vi "Alignment Offset SLM.vi"() -> (3 "number of steps align":u16)   [LabVIEW 2014]
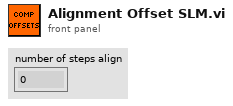
[diagram p1: front panel]
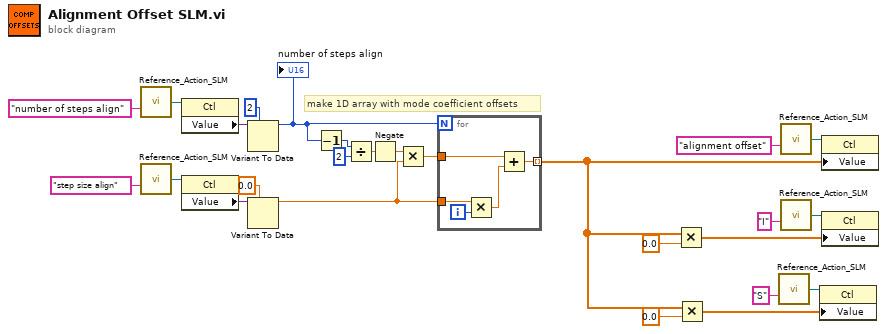
[diagram p0: block diagram]
diagram:
  # "make 1D array with mode coefficient offsets"
  n1 = call "Reference_Action_SLM.vi"("Control Name"="number of steps align") -> ("Ref OUT"=w15:refnum<vi>)  [unwired: 12 in, 2 out]
  n2 = call "Reference_Action_SLM.vi"("Control Name"="step size align") -> ("Ref OUT"=w20:refnum<vi>)  [unwired: 12 in, 2 out]
  n3 = property class="Ctl"(reference=w15) -> ("Value"=w16:variant)  [unwired: 1 in, 2 out]
  n4 = property class="Ctl"(reference=w20) -> ("Value"=w21:variant)  [unwired: 1 in, 2 out]
  n5 = Variant To Data(type=u16 2 ("y"), Variant=w16) -> (data=w12:u16)  [unwired: 1 in, 1 out]
  "number of steps align" <- w12
  n6 = Variant To Data(type=0.0 ("x*y"), Variant=w21) -> (data=w18:dbl)  [unwired: 1 in, 1 out]
  n7 = Decrement(x=w12) -> (x-1=w26:u16)
  n8 = Divide(x=w26, y=u16 2) -> (x/y=w24:dbl)
  n9 = Negate(x=w24) -> (-x=w25:dbl)
  n10 = Multiply(x=w25, y=w18) -> (x*y=w22:dbl)
  n11 = for {
    N: w12 -> [_]
    tunnel: w18 -> [w29]
    tunnel: w22 -> [w31]
    tunnel: [w27] -> w3 mode=indexing
    i -> [w30]
    n12 = Multiply(x=w29, y=w30) -> (x*y=w28:dbl)
    n13 = Add(x=w31, y=w28) -> (x+y=w27:dbl)
  }
  n14 = Multiply(x=w3, y=0.0) -> (x*y=w5:dbl[])
  n15 = Multiply(x=w3, y=0.0) -> (x*y=w4:dbl[])
  n16 = call "Reference_Action_SLM.vi"("Control Name"="S") -> ("Ref OUT"=w8:refnum<vi>)  [unwired: 12 in, 2 out]
  n17 = call "Reference_Action_SLM.vi"("Control Name"="alignment offset") -> ("Ref OUT"=w11:refnum<vi>)  [unwired: 12 in, 2 out]
  n18 = call "Reference_Action_SLM.vi"("Control Name"="I") -> ("Ref OUT"=w9:refnum<vi>)  [unwired: 12 in, 2 out]
  n19 = property class="Ctl"(reference=w8, "Value"=w4) -> ()  [unwired: 1 in, 2 out]
  n20 = property class="Ctl"(reference=w11, "Value"=w3) -> ()  [unwired: 1 in, 2 out]
  n21 = property class="Ctl"(reference=w9, "Value"=w5) -> ()  [unwired: 1 in, 2 out]
